vi "Test_HSDIO_AWG_Standalone.vi"(8 "error in (no error)":errorcluster) -> (0 "error out":errorcluster)   [LabVIEW 2017]
doc: "This VI inits a waveform generation session for AWG-5421. This is a basic example that shows how to setup the board in order to generate waveforms according to a script. \nBy default this configuration uses one channel CH0, and one script trigger ScriptTrigger0. The ScriptTrigger0 is waiting for an external trigger : i.e. a digital Edge on pin PFI 0 by default.\n\nThere are various options for the script to be used. Consult the Script control help for more information on configuring the example for specific scripts."
uses:
  controls/HSDIO_6541_Inputs.ctl
  <instrlib>/niHSDIO/niHSDIO.llb/niHSDIO_ctl Trigger Source Values (Ring).ctl
  controls/SOFTWARE_Inputs.ctl
  controls/TIMING_Inputs.ctl
panel:
  in  "TIMING Inputs":T1={"Number of Acquisitions "=1, "Number of Accumulations"=1, "Table of Waveforms"=[], "Script Text"=""} caption="SEQUENCE Inputs" {"Number of Accumulations" min=0 max=50 step=1; "Number of Acquisitions" min=1 max=10 step=1}
  out "FIFO used":i64
  in  "Use Software Trigger":bool=TRUE
  in  "SOFTWARE Inputs":T2={"Application Directory"=path "D:/S.O.F.T.S/LABVIEW/PIL", "Software Version"="1.0.0", "Data Path"=path "D:/PIRENEA/DATA", "XML Path"=path "D:/PIRENEA/DATA", "XML File Filter"="*.xml", "XML Saved Path"=path "D:/S.O.F.T.S/LABVIEW/PIL/resources", "Excit Scripts Path"=path "D:/PIRENEA/EXCIT_SCRIPTS", "Excit Scripts File Filter"="*.txt", "Excit Waveforms Path"=path "D:/PIRENEA/EXCIT_WFMS", "Excit Waveforms File Filter"="*.bin", "Timing Scripts Path"=path "D:/PIRENEA/TIMING_SCRIPTS", "Timing Scripts File Filter"="*.txt", "Timing Waveforms Path"=path "D:/PIRENEA/TIMING_WFMS", "Timing Waveforms File Filter"="*.bin", "Trapping Waveforms Path"=path "D:/PIRENEA/TRAPPING_WFMS", "Trapping Waveforms File Filter"="*.bin"}
  in  "HSDIO 6541 Inputs":T3={"Resource Name"="HSDIO_6541", "Clock Rate"=1000000.0, "Trigger Source"="PFI0"} {"Clock Rate" format="%.2p"}
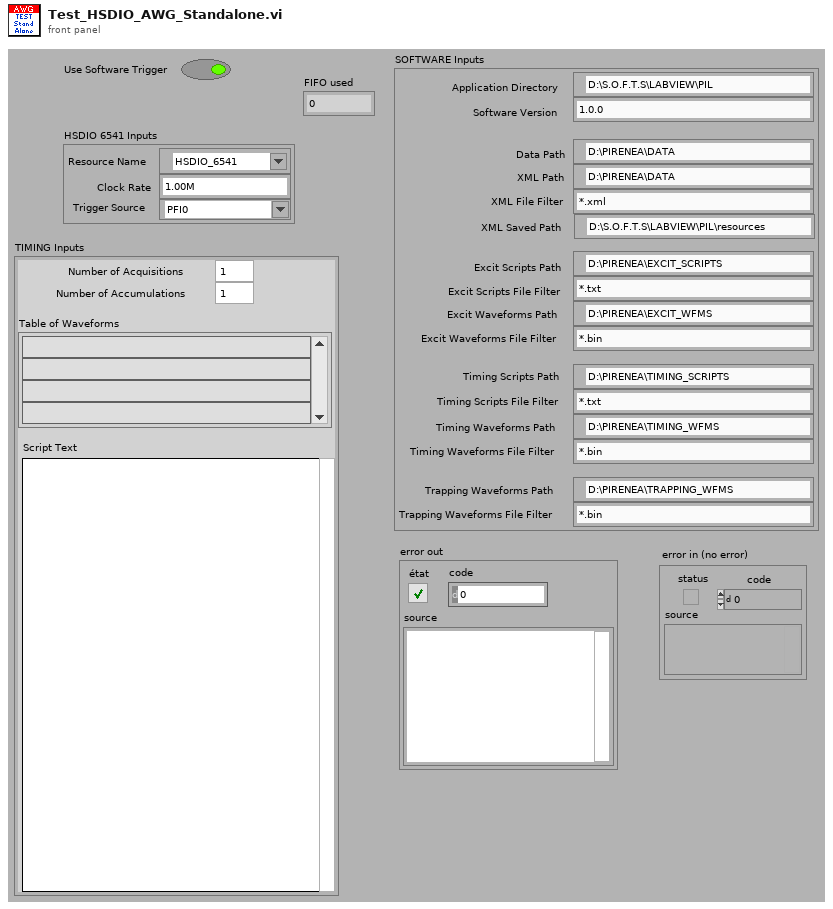
[diagram p1: front panel]
types:
  T1 = typedef "TIMING_Inputs.ctl" = cluster{"Number of Acquisitions ":i16, "Number of Accumulations":i16, "Table of Waveforms":string[], "Script Text":string}
  T2 = typedef "SOFTWARE_Inputs.ctl" = cluster{"Application Directory":path, "Software Version":string, "Data Path":path, "XML Path":path, "XML File Filter":string, "XML Saved Path":path, "Excit Scripts Path":path, "Excit Scripts File Filter":string, "Excit Waveforms Path":path, "Excit Waveforms File Filter":string, "Timing Scripts Path":path, "Timing Scripts File Filter":string, "Timing Waveforms Path":path, "Timing Waveforms File Filter":string, "Trapping Waveforms Path":path, "Trapping Waveforms File Filter":string}
  T3 = typedef "HSDIO_6541_Inputs.ctl" = cluster{"Resource Name":refnum<k15>, "Clock Rate":dbl, "Trigger Source":T4}
  T4 = typedef "niHSDIO_ctl Trigger Source Values (Ring).ctl" = string
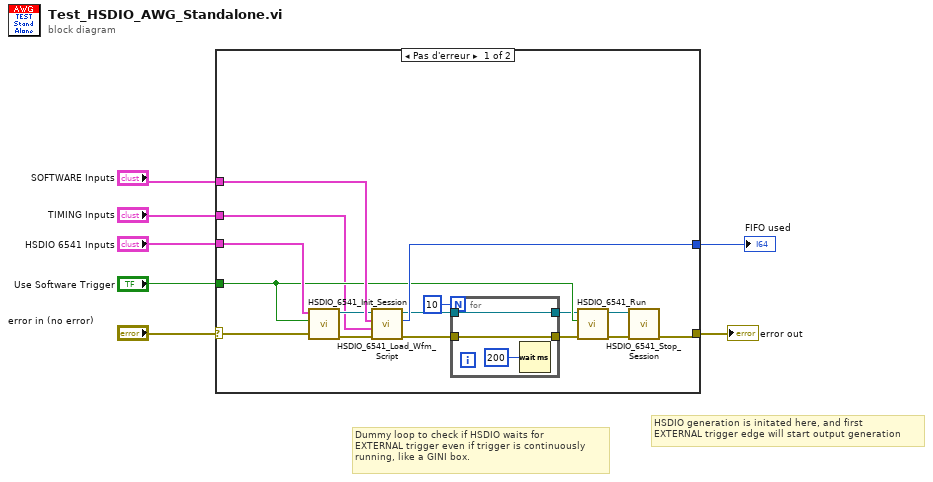
[diagram p0: block diagram]
diagram:
  # "HSDIO generation is initated here, and first\nEXTERNAL trigger edge will start output generation"
  # "Dummy loop to check if HSDIO waits for\nEXTERNAL trigger even if trigger is continuously\nrunning, like a GINI box."
  n1 = case shown="Pas d'erreur" "error in (no error)" {
    selector: "error in (no error)" -> [w16 w27]
    tunnel: [w23 w27] -> w7
    tunnel: "HSDIO 6541 Inputs" -> [w22 _]
    tunnel: "SOFTWARE Inputs" -> [w20 _]
    tunnel: "Use Software Trigger" -> [w14 _]
    tunnel: [w15 _] -> w2
    tunnel: "TIMING Inputs" -> [w8 _]
    frame No Error {
      n2 = call "HSDIO_6541_Init_Session.vi"("error in (no error)"=w16, "Use Software Trigger"=w14, "HSDIO 6541 Inputs"=w22) -> ("error out"=w21:errorcluster, "instrument handle out"=w19:refnum<k15>)  [unwired: 7 in]
      n3 = call "HSDIO_6541_Load_Wfm_Script.vi"("error  in"=w21, "TIMING Inputs"=w8, "SOFTWARE Inputs"=w20, "instrument handle in"=w19) -> ("error out"=w11:errorcluster, "FIFO used"=w15:i64, "instrument handle out"=w13:refnum<k15>)  [unwired: 4 in, 1 out]
      n4 = for {
        N: 10 -> [_]
        tunnel: w13 -> [w26]
        tunnel: [w26] -> w12
        tunnel: w11 -> [w25]
        tunnel: [w25] -> w10
        n5 = Wait (ms)(milliseconds to wait=u32 200 ("attente (ms)")) -> ()  [unwired: 1 out]
      }
      n6 = call "HSDIO_6541_Run.vi"("error  in"=w10, "Use Software trigger"=w14, "instrument handle in"=w12) -> ("error out"=w17:errorcluster, "instrument handle out"=w18:refnum<k15>)  [unwired: 7 in]
      n7 = call "HSDIO_6541_Stop_Session.vi"("error in (no error)"=w17, "instrument handle in"=w18) -> ("error out"=w23:errorcluster)  [unwired: 9 in]
    }
    frame Error {
    }
  }
  "error out" <- w7
  "FIFO used" <- w2
